vi "Insert New Path.vi"(9 "Browse Dir Ref":refnum<vi> caption="浏览目录引用", 10 "Editing Path Ref":refnum<vi> caption="编辑路径引用", 11 "Include Paths Ref":refnum<vi> caption="包括路径引用") -> (1 "Row Number":i32 caption="行数", 2 "Path Strings Out":T1 caption="路径字符串输出", 3 "Dup Include Paths Ref":refnum<vi> caption="包括路径引用副本")   [LabVIEW 2011, in "NISAST Include Paths.xctl"]
uses:
  NISAST Include Paths.xctl
  Data.ctl
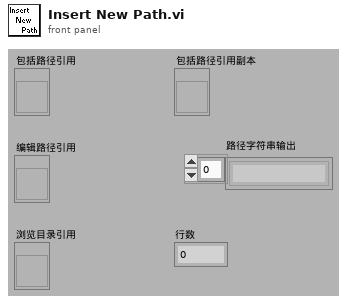
[diagram p1: front panel]
types:
  T1 = typedef "NISAST Include Paths.xctl/Data.ctl" = string[]
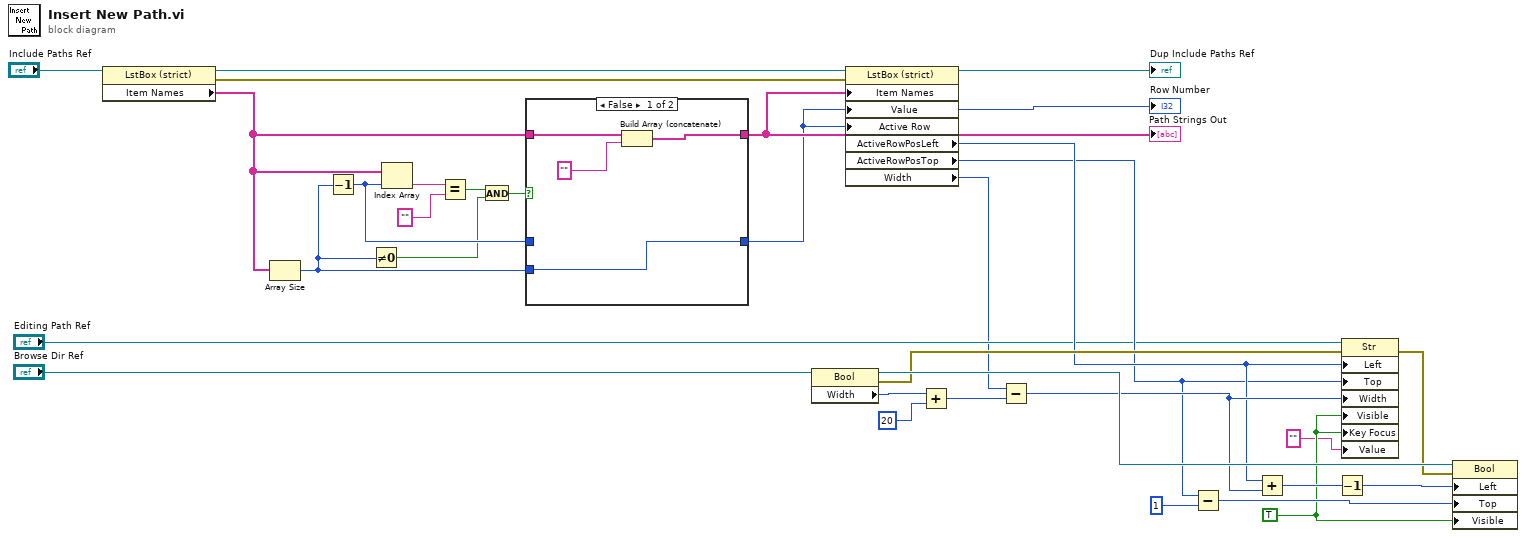
[diagram p0: block diagram]
diagram:
  w12 = TRUE ("Visible")
  n1 = property class="LstBox (strict)"(reference="Include Paths Ref") -> (reference out=w32:refnum<vi>, error out=w29:errorcluster, "Item Names"=w28:string[])  [unwired: 1 in]
  n2 = Array Size(array=w28) -> (size(s)=w4:i32)
  n3 = Decrement(x=w4) -> (x-1=w24:i32)
  n4 = Not Equal To 0?(x=w4) -> (x != 0?=w1:bool)
  n5 = Index Array(array=w28, index=w24) -> (element=w27:string)
  n6 = Equal?(x=w27, y="") -> (x = y?=w3:bool)
  n7 = And(x=w3, y=w1) -> (x .and. y?=w2:bool)
  n8 = case shown="False" w2 {
    tunnel: [w35 w37] -> w25
    tunnel: w28 -> [w34 w37]
    tunnel: [w33 w38] -> w23
    tunnel: w4 -> [w33 _]
    tunnel: w24 -> [_ w38]
    frame False {
      n9 = Build Array (concatenate)(w34, "") -> (w35:string[])
    }
    frame True {
    }
  }
  "Path Strings Out" <- w25
  "Row Number" <- w23
  n10 = property class="Bool"(reference="Browse Dir Ref") -> (reference out=w22:refnum<vi>, error out=w11:errorcluster, "Width"=w19:u32)  [unwired: 1 in]
  n11 = property class="LstBox (strict)"(reference=w32, error in=w29, "Item Names"=w25, "Value"=w23, "Active Row"=w23) -> (reference out=→"Dup Include Paths Ref":refnum<vi>, "ActiveRowPosLeft"=w10:i32, "ActiveRowPosTop"=w9:i32, "Width"=w6:u32)  [unwired: 1 out]
  n12 = Add(x=w19, y=u32 20) -> (x+y=w18:u32)
  n13 = Subtract(x=w6, y=w18) -> (x-y=w21:u32)
  n14 = Subtract(x=w9, y=u32 1) -> (x-y=w16:u32)
  n15 = Add(x=w10, y=w21) -> (x+y=w14:u32)
  n16 = Decrement(x=w14) -> (x-1=w13:u32)
  n17 = property class="Str"(reference="Editing Path Ref", error in=w11, "Left"=w10, "Top"=w9, "Width"=w21, "Visible"=w12, "Key Focus"=w12, "Value"="") -> (error out=w17:errorcluster)  [unwired: 1 out]
  n18 = property class="Bool"(reference=w22, error in=w17, "Left"=w13, "Top"=w16, "Visible"=w12) -> ()  [unwired: 2 out]
